vi "machine control.vi"() -> ()   [LabVIEW 2018]
uses:
  ctl/state machine.ctl
  ctl/state machine_read waveform.ctl
  <vilib>/Utility/file.llb/Write To Spreadsheet File (string).vi
panel:
  out "error out":errorcluster
  out "Channel detail information":string[](array[string])
  in  "Convert Y unit to voltage":bool=TRUE
  out "Log":string
  in  "Stop LabVIEW":bool
  out "Last read waveform time(ms)":u32
  in  "Interval(ms)":u32=2000 min=2000 step=100
  in  "Read waveform(continuous)":bool
  in  "CH2":T1
  in  "CH1":T2
  in  "Syntax Testing":cluster{"Syntax":string, "Send":bool}={"Syntax"="*IDN?", "Send"=FALSE}
  in  "Save XY graph":bool
  out "XY Graph":cluster{dbl[], dbl[]}[](graph)
  out "Read buffer":string
  in  "Get instrument information":bool
  in  "Read waveform(single)":bool
  in  "Horizontal scale(TIME/DIV)":T3(ring)
  in  "Autoset":bool
  in  "Device":refnum<visa-resource-name>
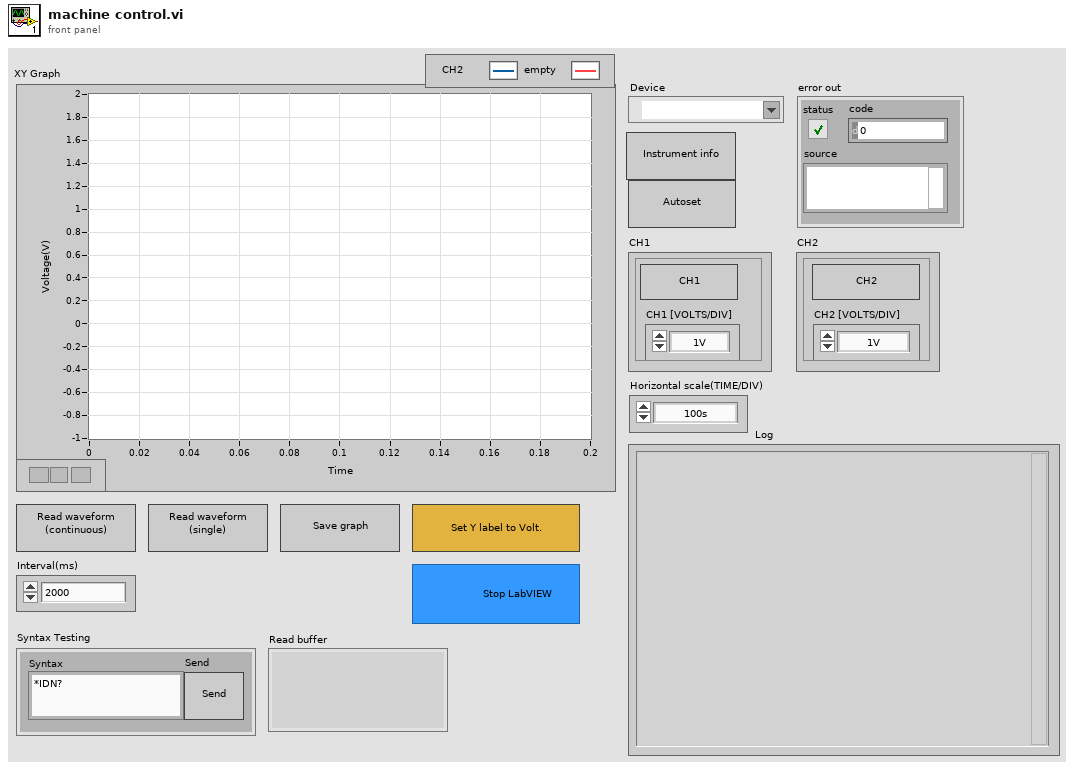
[diagram p1: front panel]
types:
  T1 = cluster{"Enable CH2":bool, "CH2 [VOLTS/DIV]":enum16{"1V", "500mV", "200mV", "100mV", "50mV", "20mV", "10mV", "5mV", "2mV"}}
  T2 = cluster{"Enable CH1":bool, "CH1 [VOLTS/DIV]":enum16{"1V", "500mV", "200mV", "100mV", "50mV", "20mV", "10mV", "5mV", "2mV"}}
  T3 = enum16{"100s", "50s", "20s", "10s", "5s", "2s", "1s", "500ms", "200ms", "100ms", "50ms", "20ms", "10ms", "5ms", "2ms", "1ms", "500£gs", "200£gs ", "100£gs ", "50£gs ", "20£gs ", "10£gs ", "5£gs ", "2£gs", "1£gs", "500ns", "200ns", "100ns", "50ns", "20ns", "10ns", "5ns", "2ns", "1ns"}
  T4 = typedef "state machine.ctl" = enum16{"Initialize", "Open VISA", "Run", "Close VISA"}
  T5 = typedef "state machine_read waveform.ctl" = enum16{"Read waveform", "Data parsing", "Plot graph"}
  T6 = enum16{"1V", "500mV", "200mV", "100mV", "50mV", "20mV", "10mV", "5mV", "2mV"}
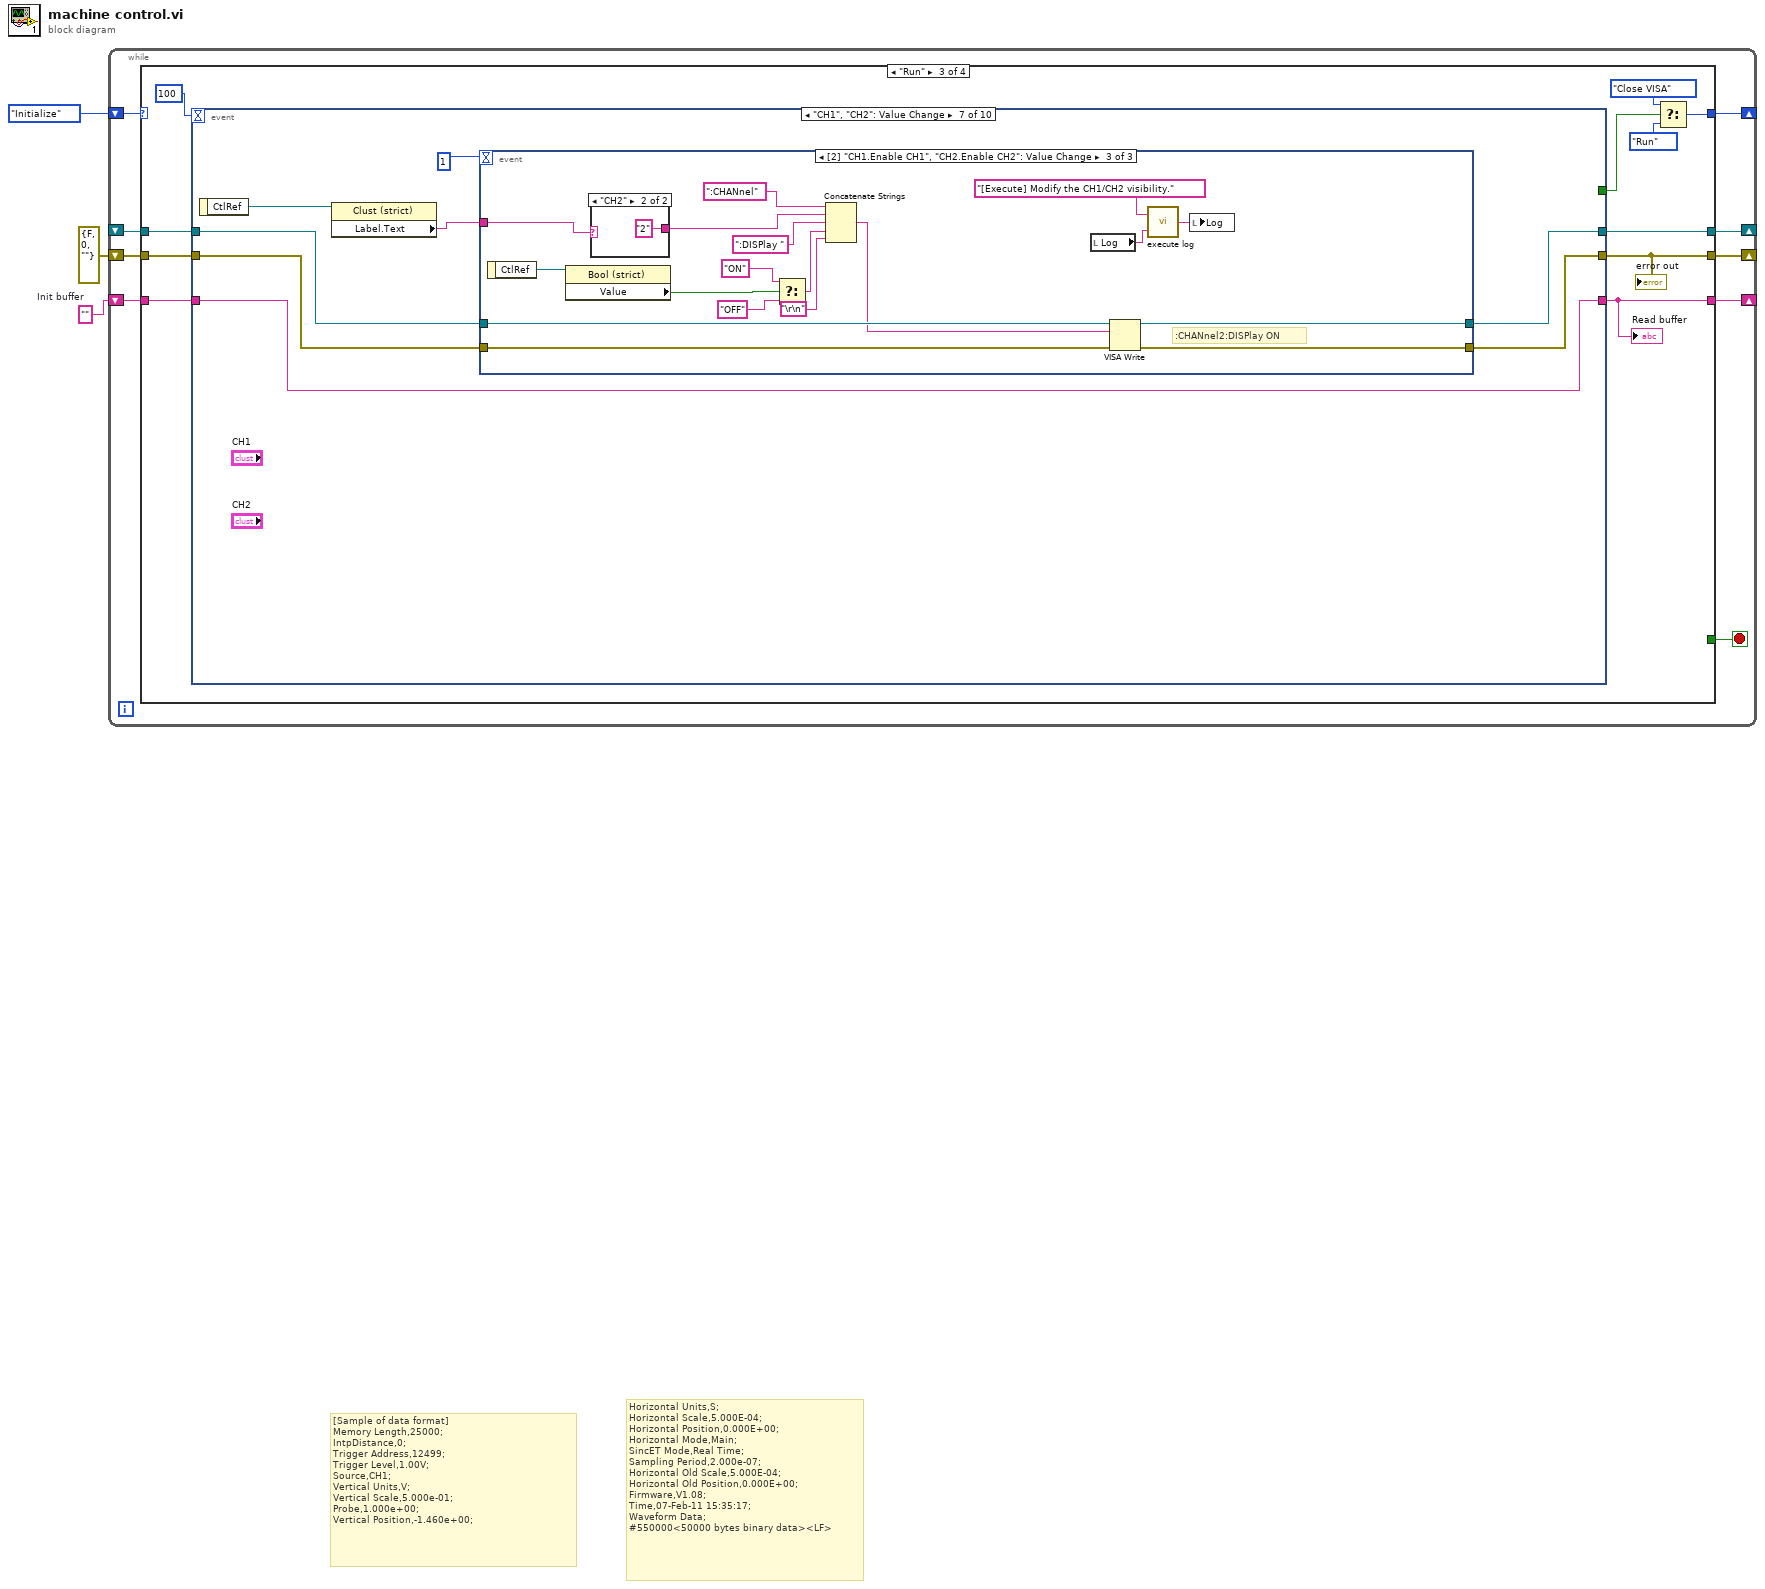
[diagram p0: block diagram]
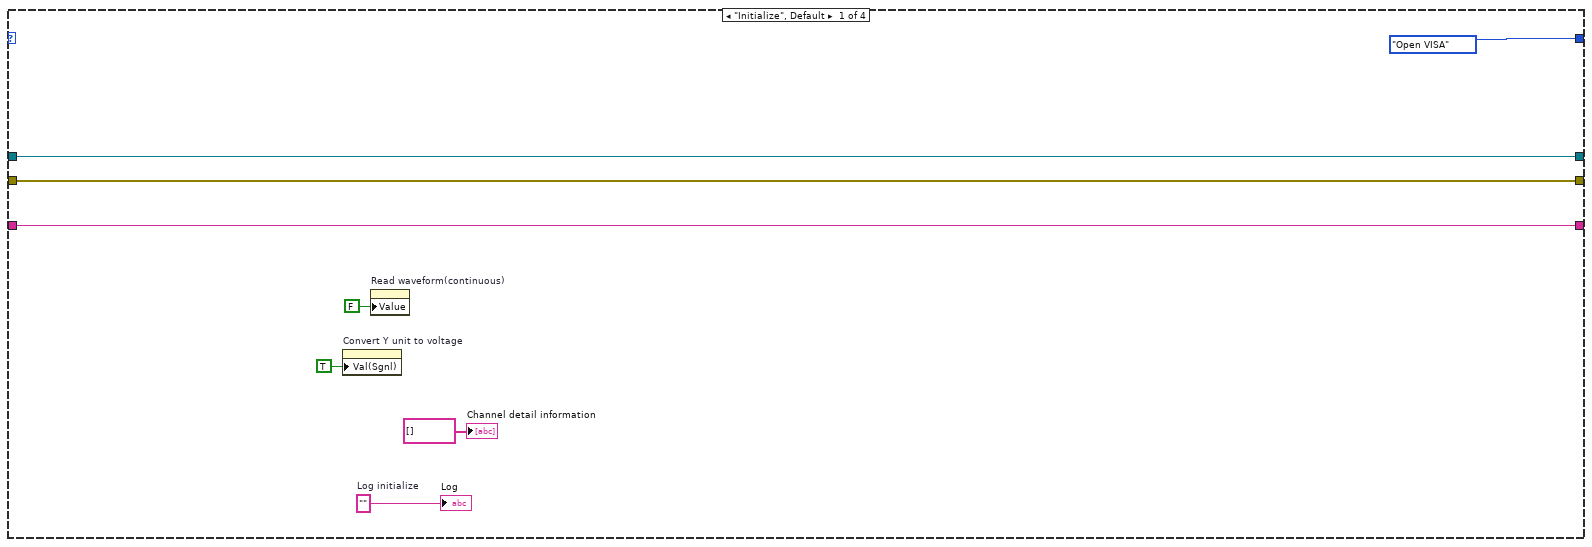
[diagram p2: hidden frame]
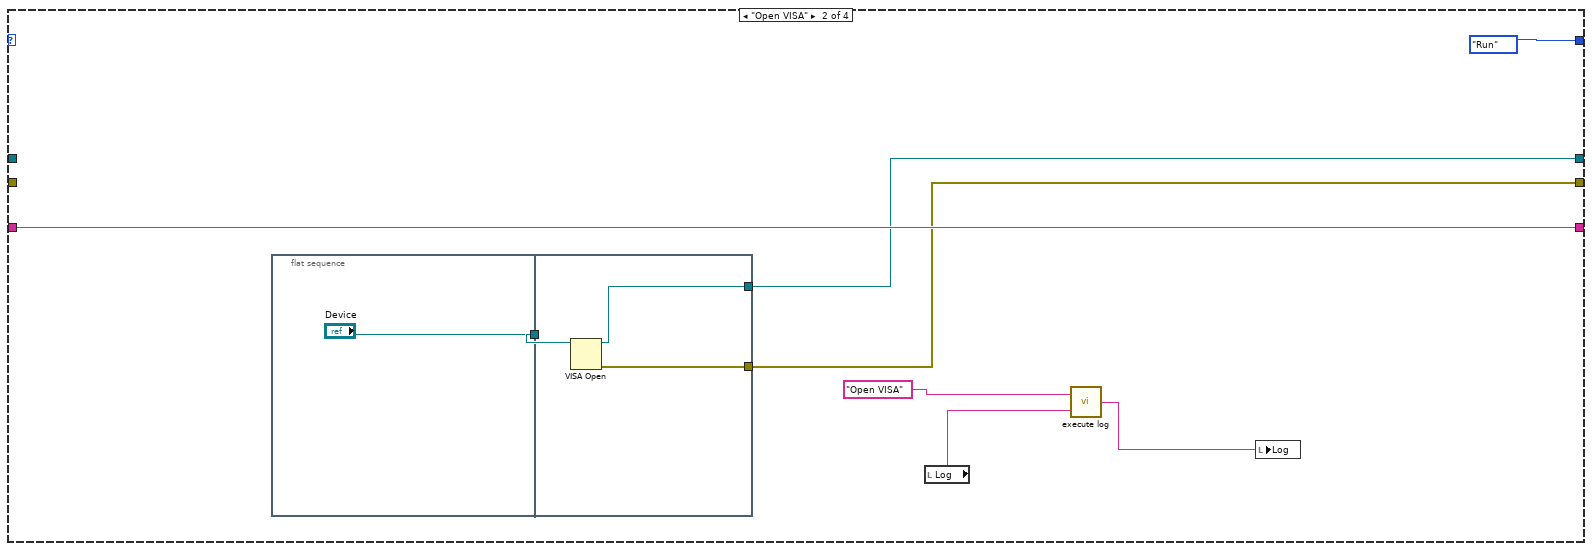
[diagram p3: hidden frame]
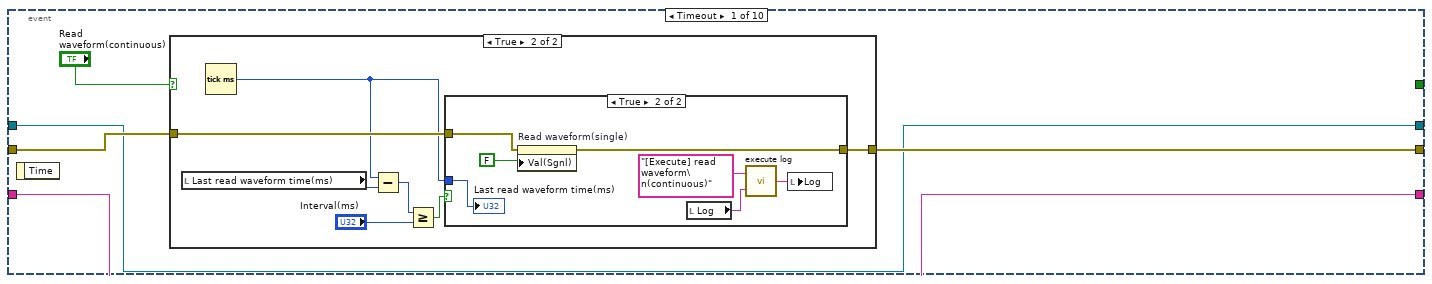
[diagram p4: hidden frame]
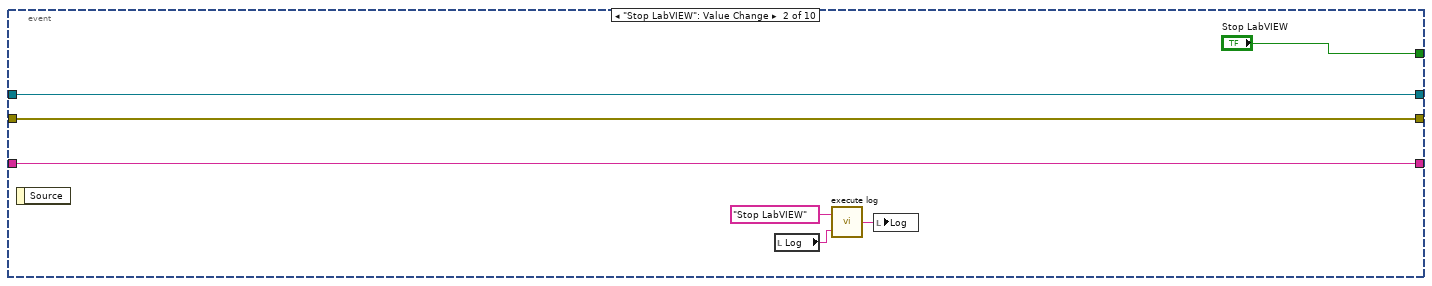
[diagram p7: hidden frame]
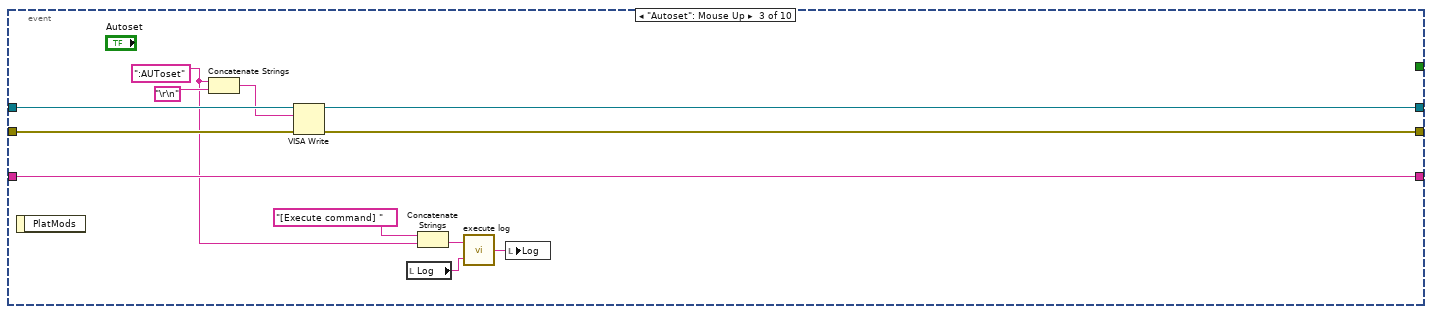
[diagram p8: hidden frame]
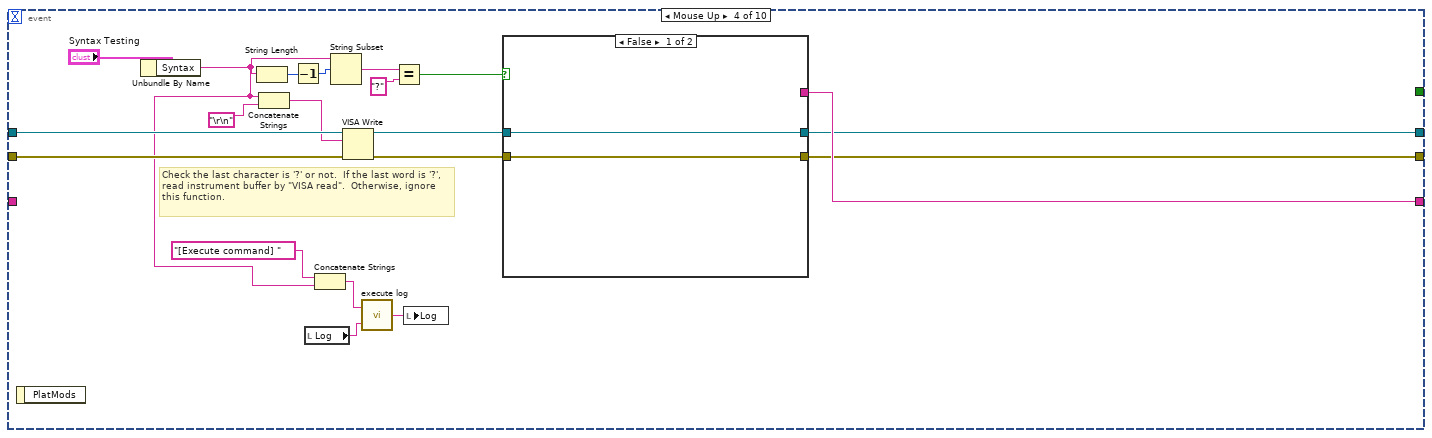
[diagram p9: hidden frame]
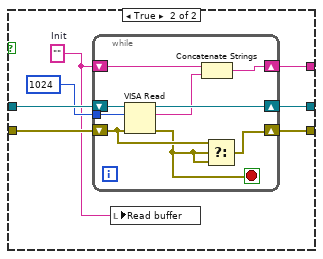
[diagram p10: hidden frame]
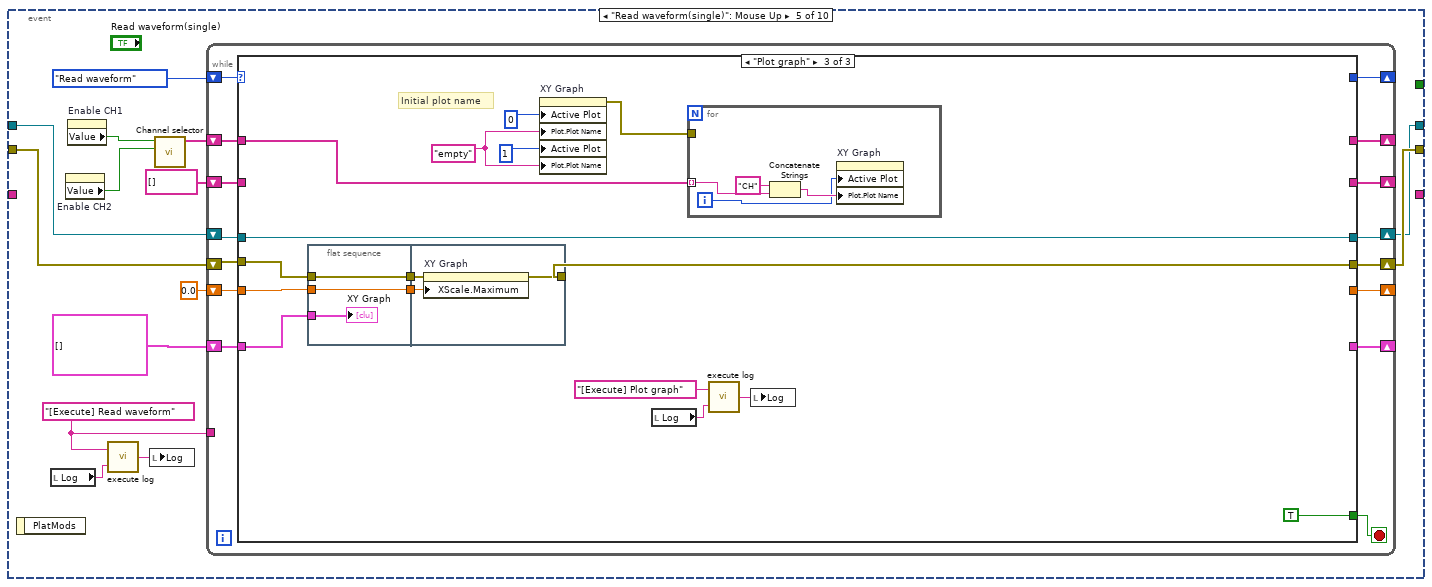
[diagram p11: hidden frame]
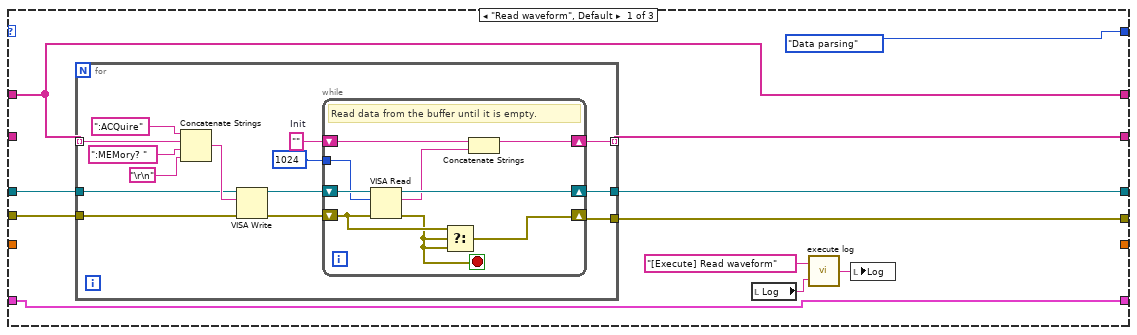
[diagram p12: hidden frame]
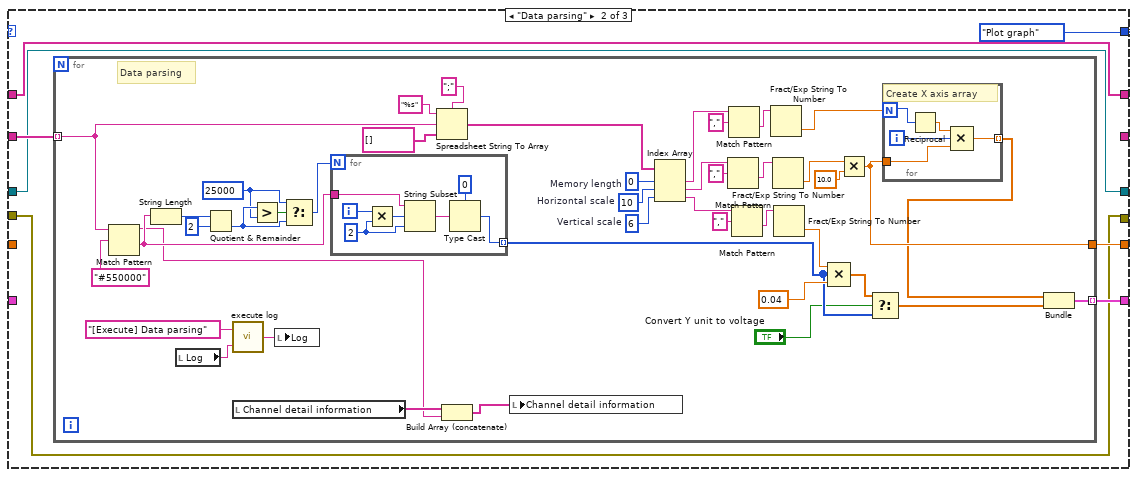
[diagram p13: hidden frame]
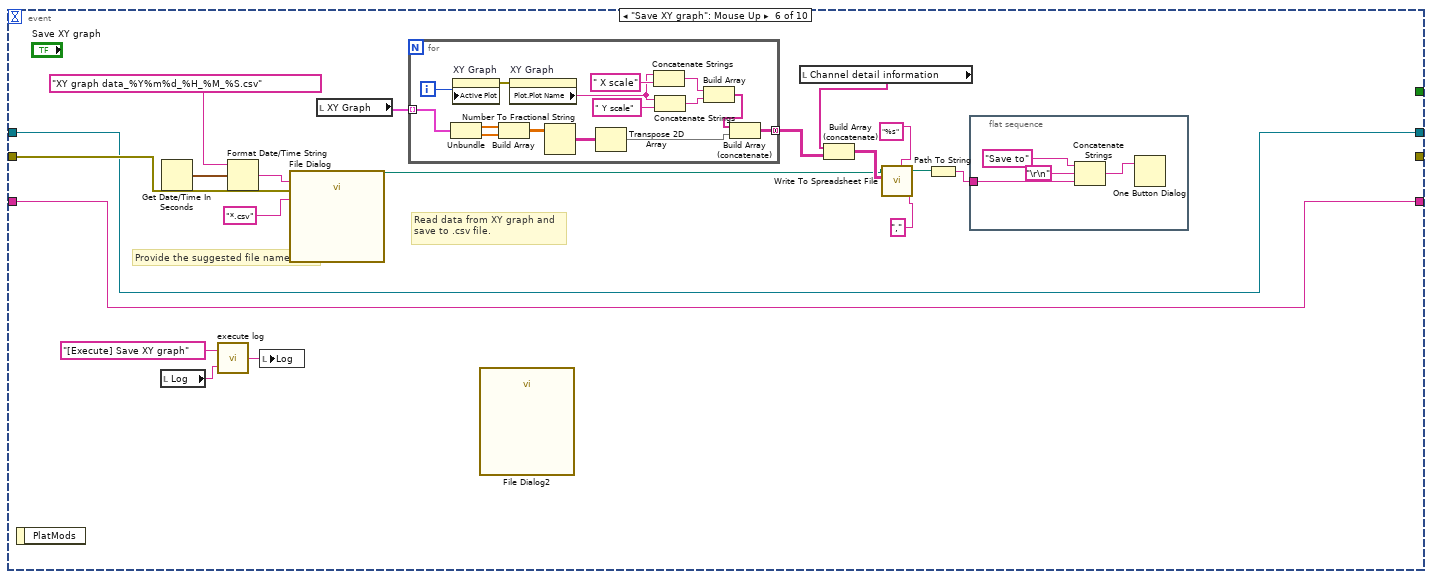
[diagram p14: hidden frame]
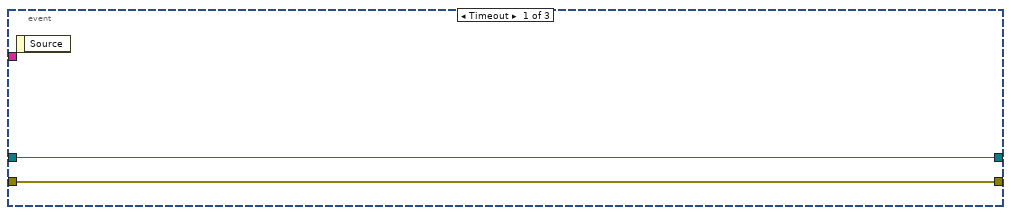
[diagram p15: hidden frame]
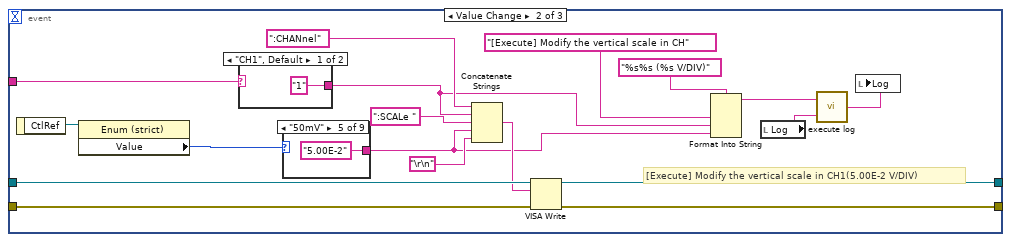
[diagram p16: hidden frame]
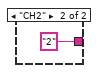
[diagram p17: hidden frame]
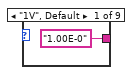
[diagram p18: hidden frame]
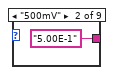
[diagram p19: hidden frame]
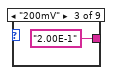
[diagram p20: hidden frame]
diagram:
  w2 = ""  # Init buffer
  # "Horizontal Units,S;\nHorizontal Scale,5.000E-04;\nHorizontal Position,0.000E+00;\nHorizontal Mode,Main;\nSincET Mode,Real Time;\nSampling Period,2.000e-07;\nHorizontal Old Scale,5.000E-04;\nHorizontal Old Position,0.000E+00;\nFirmware,V1.08;\nTime,07-Feb-11 15:35:17;\nWaveform Data;\n#550000<50000 bytes binary data><LF>"
  # "[Sample of data format]\nMemory Length,25000;\nIntpDistance,0;\nTrigger Address,12499;\nTrigger Level,1.00V;\nSource,CH1;\nVertical Units,V;\nVertical Scale,5.000e-01;\nProbe,1.000e+00;\nVertical Position,-1.460e+00;"
  n1 = while {
    shift-right: [w11] -> _
    shift-left: state_machine."Initialize" -> [w12]
    shift-right: [w8] -> _
    shift-left: w2 -> [w5]
    shift-right: [w9] -> _
    shift-left: _ -> [w6]
    shift-right: [w10] -> _
    shift-left: errorcluster {"status"=FALSE, "code"=0, "source"=""} ("error out") -> [w7]
    stop <- w4 stop-if-true
    n2 = case shown="\"Run\"" w12 {
      tunnel: [state_machine."Open VISA" state_machine."Run" w33 _] -> w11
      tunnel: [w17 w21 w43 w442] -> w10
      tunnel: [w18 w22 w42 _] -> w9
      tunnel: [w19 w27 w41 w443] -> w8
      tunnel: w7 -> [w17 _ w40 w444]
      tunnel: w6 -> [w18 _ w39 w445]
      tunnel: w5 -> [w19 w27 w38 w443]
      tunnel: [_ _ _ TRUE] -> w4
      frame "Initialize", Default {
        w14 = ""  # Log initialize
        n3 = property on="Convert Y unit to voltage" class="Bool (strict)"("Val(Sgnl)"=TRUE ("Read waveform(continuous)")) -> ()  [unwired: 2 in, 2 out]
        n4 = property on="Read waveform(continuous)" class="Bool (strict)"("Value"=FALSE ("Read waveform(continuous)")) -> ()  [unwired: 2 in, 2 out]
        "Log" <- w14
        "Channel detail information" <- string[] [] ("Channel detail information")
      }
      frame "Open VISA" {
        n5 = flat-sequence {
          tunnel: ["Device"] -> w23
          tunnel: w23 -> [w32]
          tunnel: [w31] -> w22
          tunnel: [w30] -> w21
          frame #0 {
          }
          frame #1 {
            n6 = VISA Open(VISA resource name=w32) -> (VISA resource name=w31:refnum<visa-resource-name>, error out=w30:errorcluster)  [unwired: 4 in]
          }
        }
        n7 = local read "Log"() -> (w24:string)
        n8 = call "execute log.vi"("log window"=w24, "input string"="Open VISA") -> ("output string"=w25:string)
        n9 = local write "Log"(w25) -> ()
      }
      frame "Run" {
        n10 = event shown="[6] \"CH1\", \"CH2\": Value Change" {
          selector: _ -> [_ _ _ _ _ _ _ _ _ _]
          dyn-events: _ -> [_ _ _ _ _ _ _ _ _ _]
          timeout: 100 -> [_ _ _ _ _ _ _ _ _ _]
          tunnel: w39 -> [w45 w70 w83 w95 w130 w288 w315 w383 w386 w400]
          tunnel: w40 -> [w47 w71 w82 w92 w129 w289 w316 w382 w385 w399]
          tunnel: [w44 w69 w77 w96 _ w290 w311 w377 w384 w394] -> w41
          tunnel: [w45 w70 w81 w94 w124 w288 w318 w379 w386 w398] -> w42
          tunnel: [w46 w71 w80 w93 w125 _ w317 w378 w385 w397] -> w43
          tunnel: [_ "Stop LabVIEW" _ _ _ _ _ _ _ _] -> w36
          tunnel: w38 -> [w44 w69 w77 _ _ w290 w311 _ w384 w394]
          event Timeout {
            n11 = event-data() -> ()  [unwired: 1 in, 1 out]
            n12 = case shown="True" "Read waveform(continuous)" {
              tunnel: w47 -> [w49 w52]
              tunnel: [w49 w51] -> w46
              frame False {
              }
              frame True {
                n13 = local read "Last read waveform time(ms)"() -> (w56:u32)
                n14 = Tick Count (ms)() -> (millisecond timer value=w50:u32)
                n15 = Subtract(x=w50, y=w56) -> (x-y=w53:u32)
                n16 = Greater Or Equal?(x=w53, y="Interval(ms)") -> (x >= y?=w54:bool)
                n17 = case shown="True" w54 {
                  tunnel: w52 -> [w57 w59]
                  tunnel: [w57 w64] -> w51
                  tunnel: w50 -> [_ w60]
                  frame False {
                    # "Nothing"
                  }
                  frame True {
                    n18 = property on="Read waveform(single)" class="Bool (strict)"(error in=w59, "Val(Sgnl)"=FALSE) -> (error out=w64:errorcluster)  [unwired: 1 in, 1 out]
                    n19 = local read "Log"() -> (w61:string)
                    n20 = call "execute log.vi"("log window"=w61, "input string"="[Execute] read waveform\n(continuous)") -> ("output string"=w62:string)
                    n21 = local write "Log"(w62) -> ()
                    "Last read waveform time(ms)" <- w60
                  }
                }
              }
            }
          }
          event "Stop LabVIEW": Value Change {
            n22 = event-data() -> ()  [unwired: 1 in, 1 out]
            n23 = local read "Log"() -> (w65:string)
            n24 = call "execute log.vi"("log window"=w65, "input string"="Stop LabVIEW") -> ("output string"=w66:string)
            n25 = local write "Log"(w66) -> ()
          }
          event "Autoset": Mouse Up {
            w74 = ":AUToset"
            n26 = event-data() -> ()  [unwired: 1 in, 1 out]
            n27 = Concatenate Strings(w74, "\r\n") -> (w79:string)
            n28 = VISA Write(VISA resource name=w83, write buffer=w79, error in (no error)=w82) -> (VISA resource name out=w81:refnum<visa-resource-name>, error out=w80:errorcluster)  [unwired: 1 out]
            n29 = local read "Log"() -> (w75:string)
            n30 = Concatenate Strings("[Execute command] " ("input string"), w74) -> (w72:string)
            n31 = call "execute log.vi"("log window"=w75, "input string"=w72) -> ("output string"=w76:string)
            n32 = local write "Log"(w76) -> ()
          }
          event "Syntax Testing.Send": Mouse Up {
            # "Check the last character is '?' or not.  If the last word is '?', read instrument buffer by \"VISA read\".  Otherwise, ignore this function."
            n33 = event-data() -> ()  [unwired: 1 in, 1 out]
            n34 = Unbundle By Name("Syntax Testing") -> ("Syntax"=w85:string)
            n35 = String Length(string=w85) -> (length=w98:i32)
            n36 = Concatenate Strings(w85, "\r\n") -> (w90:string)
            n37 = Decrement(x=w98) -> (x-1=w99:i32)
            n38 = local read "Log"() -> (w87:string)
            n39 = Concatenate Strings("[Execute command] " ("input string"), w85) -> (w86:string)
            n40 = String Subset(string=w85, offset (0)=w99) -> (substring=w100:string)  [unwired: 1 in]
            n41 = VISA Write(VISA resource name=w95, write buffer=w90, error in (no error)=w92) -> (VISA resource name out=w103:refnum<visa-resource-name>, error out=w102:errorcluster)  [unwired: 1 out]
            n42 = call "execute log.vi"("log window"=w87, "input string"=w86) -> ("output string"=w88:string)
            n43 = Equal?(x=w100, y="?") -> (x = y?=w97:bool)
            n44 = local write "Log"(w88) -> ()
            n45 = case shown="False" w97 {
              tunnel: w103 -> [w105 w112]
              tunnel: [w105 w111] -> w94
              tunnel: w102 -> [w104 w110]
              tunnel: [w104 w109] -> w93
              tunnel: [_ w107] -> w96
              frame False {
              }
              frame True {
                w106 = ""  # Init
                n46 = while {
                  tunnel: u32 1024 ("byte count") -> [w119]
                  shift-right: [w120] -> w111
                  shift-left: w112 -> [w121]
                  shift-right: [w116] -> w109
                  shift-left: w110 -> [w115]
                  shift-right: [w117] -> w107
                  shift-left: w106 -> [w114]
                  stop <- w113 stop-if-true
                  n47 = VISA Read(VISA resource name=w121, byte count=w119, error in (no error)=w115) -> (VISA resource name out=w120:refnum<visa-resource-name>, read buffer=w118:string, error out=w113:errorcluster)  [unwired: 1 out]
                  n48 = Concatenate Strings(w114, w118) -> (w117:string)
                  n49 = Select(t=w115, s=w113, f=w113) -> (s? t:f=w116:errorcluster)
                }
                n50 = local write "Read buffer"(w106) -> ()
              }
            }
          }
          event "Read waveform(single)": Mouse Up {
            w126 = "[Execute] Read waveform" ("input string")
            n51 = event-data() -> ()  [unwired: 1 in, 1 out]
            n52 = local read "Log"() -> (w127:string)
            n53 = property on="Enable CH2" class="Bool (strict)"() -> ("Value"=w131:bool)  [unwired: 2 in, 2 out]
            n54 = property on="Enable CH1" class="Bool (strict)"() -> ("Value"=w132:bool)  [unwired: 2 in, 2 out]
            n55 = call "execute log.vi"("log window"=w127, "input string"=w126) -> ("output string"=w128:string)
            n56 = local write "Log"(w128) -> ()
            n57 = call "Channel selector.vi"("CH2"=w131, "CH1"=w132) -> ("Array"=w123:string[])  [unwired: 9 in]
            n58 = while {
              shift-right: [w141] -> _
              shift-left: state_machine_read_waveform."Read waveform" -> [w150]
              shift-right: [w147] -> w124
              shift-left: w130 -> [w148]
              shift-right: [w146] -> w125
              shift-left: w129 -> [w149]
              shift-right: [w145] -> _
              shift-left: string[] [] -> [w144]
              shift-right: [w143] -> _
              shift-left: cluster{dbl[], dbl[]}[] [] -> [w140]
              shift-right: [w142] -> _
              shift-left: 0.0 -> [w139]
              tunnel: w126 -> [_]
              shift-right: [w136] -> _
              shift-left: w123 -> [w137]
              stop <- w138 stop-if-true
              n59 = case shown="\"Plot graph\"" w150 {
                tunnel: w149 -> [w161 w186 w259]
                tunnel: w148 -> [w160 w187 w255]
                tunnel: [w159 w187 w255] -> w147
                tunnel: [w158 w186 w257] -> w146
                tunnel: [w157 _ _] -> w145
                tunnel: w144 -> [_ w191 _]
                tunnel: [w152 w190 _] -> w143
                tunnel: [_ w189 _] -> w142
                tunnel: [state_machine_read_waveform."Data parsing" state_machine_read_waveform."Plot graph" _] -> w141
                tunnel: w140 -> [w152 _ w262]
                tunnel: w139 -> [_ _ w261]
                tunnel: [_ _ TRUE] -> w138
                tunnel: w137 -> [w151 w185 w247]
                tunnel: [w151 w185 _] -> w136
                frame "Read waveform", Default {
                  n60 = for {
                    tunnel: w161 -> [w167]
                    tunnel: w160 -> [w166]
                    tunnel: [w165] -> w159
                    tunnel: [w164] -> w158
                    tunnel: [w163] -> w157 mode=indexing
                    tunnel: w151 -> [w162] mode=indexing
                    w170 = ""  # Init
                    n61 = Concatenate Strings(":ACQuire", w162, ":MEMory? ", "\r\n") -> (w169:string)
                    n62 = VISA Write(VISA resource name=w166, write buffer=w169, error in (no error)=w167) -> (VISA resource name out=w173:refnum<visa-resource-name>, error out=w172:errorcluster)  [unwired: 1 out]
                    n63 = while {
                      tunnel: u32 1024 ("byte count") -> [w182]
                      shift-right: [w183] -> w165
                      shift-left: w173 -> [w184]
                      shift-right: [w179] -> w164
                      shift-left: w172 -> [w178]
                      shift-right: [w180] -> w163
                      shift-left: w170 -> [w176]
                      stop <- w177 stop-if-true
                      # "Read data from the buffer until it is empty."
                      n64 = VISA Read(VISA resource name=w184, byte count=w182, error in (no error)=w178) -> (VISA resource name out=w183:refnum<visa-resource-name>, read buffer=w181:string, error out=w177:errorcluster)  [unwired: 1 out]
                      n65 = Select(t=w178, s=w177, f=w177) -> (s? t:f=w179:errorcluster)
                      n66 = Concatenate Strings(w176, w181) -> (w180:string)
                    }
                  }
                  n67 = local read "Log"() -> (w154:string)
                  n68 = call "execute log.vi"("log window"=w154, "input string"="[Execute] Read waveform") -> ("output string"=w155:string)
                  n69 = local write "Log"(w155) -> ()
                }
                frame "Data parsing" {
                  n70 = for {
                    tunnel: w191 -> [w211] mode=indexing
                    tunnel: [w210] -> w190 mode=indexing
                    tunnel: [w209] -> w189
                    w207 = 10  # Horizontal scale
                    w208 = 6  # Vertical scale
                    w218 = 0  # Memory length
                    w214 = 25000 ("y")
                    # "Data parsing"
                    n71 = Match Pattern(string=w211, regular expression="#550000") -> (before substring=w192:string, after substring=w224:string)  [unwired: 1 in, 2 out]
                    n72 = String Length(string=w224) -> (length=w223:i32)
                    n73 = local read "Log"() -> (w197:string)
                    n74 = Quotient & Remainder(x=w223, y=2) -> (floor(x/y)=w226:i32)  [unwired: 1 out]
                    n75 = call "execute log.vi"("log window"=w197, "input string"="[Execute] Data parsing") -> ("output string"=w198:string)
                    n76 = local read "Channel detail information"() -> (w194:string[])
                    n77 = Greater?(x=w226, y=w214) -> (0:w225:bool)
                    n78 = local write "Log"(w198) -> ()
                    n79 = Select(t=w214, s=w225, f=w226) -> (s? t:f=w227:i32)
                    n80 = for {
                      N: w227 -> [_]
                      tunnel: w224 -> [w246]
                      tunnel: [w240] -> w200 mode=indexing
                      i -> [w245]
                      w243 = 2 ("length (rest)")
                      n81 = Multiply(x=w245, y=w243) -> (x*y=w244:i32)
                      n82 = String Subset(string=w246, offset (0)=w244, length (rest)=w243) -> (substring=w241:string)
                      n83 = Type Cast(type=i16 0, x=w241) -> (*(type *) &x=w240:i16)
                    }
                    n84 = Spreadsheet String To Array ("Split by ';'")(delimiter (Tab)=";", format string="%s", spreadsheet string=w211, array type (2D Dbl)=string[] [] ("Array")) -> (array=w232:string[])
                    n85 = Build Array (concatenate)(w194, w192) -> (w193:string[])
                    n86 = local write "Channel detail information"(w193) -> ()
                    n87 = Index Array(array=w232, index #1=w218, index #2=w207, index #3=w208) -> (element #1=w233:string, element #2=w206:string, element #3=w205:string)
                    n88 = Match Pattern(string=w206, regular expression=",") -> (after substring=w230:string)  [unwired: 1 in, 3 out]
                    n89 = Match Pattern(string=w233, regular expression=",") -> (after substring=w229:string)  [unwired: 1 in, 3 out]
                    n90 = Match Pattern(string=w205, regular expression=",") -> (after substring=w231:string)  [unwired: 1 in, 3 out]
                    n91 = Fract/Exp String To Number(string=w229) -> (number=w228:dbl)  [unwired: 3 in, 1 out]
                    n92 = Fract/Exp String To Number(string=w230) -> (number=w234:dbl)  [unwired: 3 in, 1 out]
                    n93 = Fract/Exp String To Number(string=w231) -> (number=w204:dbl)  [unwired: 3 in, 1 out]
                    n94 = Compound Arithmetic op=MULTIPLY(w204, w200, 0.04 ("y")) -> (w201:dbl[])
                    n95 = Multiply(x=w234, y=10.0) -> (x*y=w209:dbl)
                    n96 = Select(t=w201, s="Convert Y unit to voltage", f=w200) -> (s? t:f=w202:dbl[])
                    n97 = for {
                      N: w228 -> [w237]
                      tunnel: w209 -> [w238]
                      tunnel: [w239] -> w199 mode=indexing
                      i -> [w235]
                      # "Create X axis array"
                      n98 = Reciprocal(x=w237) -> (1/x=w236:dbl)
                      n99 = Compound Arithmetic op=MULTIPLY(w236, w235, w238) -> (w239:dbl)
                    }
                    n100 = Bundle(w199, w202) -> (w210:cluster{dbl[], dbl[]})  [unwired: 1 in]
                  }
                }
                frame "Plot graph" {
                  w248 = "empty" ("Plot.Plot Name")
                  # "Initial plot name"
                  n101 = flat-sequence {
                    tunnel: w262 -> [w269]
                    tunnel: w261 -> [w268]
                    tunnel: [w268] -> w260
                    tunnel: w259 -> [w267]
                    tunnel: [w267] -> w258
                    tunnel: w260 -> [w272]
                    tunnel: w258 -> [w271]
                    tunnel: [w270] -> w257
                    frame #0 {
                      "XY Graph" <- w269
                    }
                    frame #1 {
                      n102 = property on="XY Graph" class="XYGraph (strict)"(error in=w271, "XScale.Maximum"=w272) -> (error out=w270:errorcluster)  [unwired: 1 in, 1 out]
                    }
                  }
                  n103 = property on="XY Graph" class="XYGraph (strict)"("Active Plot"=u32 0, "Plot.Plot Name"=w248, "Active Plot"=u32 1, "Plot.Plot Name"=w248) -> (error out=w251:errorcluster)  [unwired: 2 in, 1 out]
                  n104 = local read "Log"() -> (w253:string)
                  n105 = for {
                    tunnel: w247 -> [w266] mode=indexing
                    tunnel: w251 -> [_]
                    i -> [w263]
                    n106 = Concatenate Strings("CH" ("string"), w266) -> (w264:string)
                    n107 = property on="XY Graph" class="XYGraph (strict)"("Active Plot"=w263, "Plot.Plot Name"=w264) -> ()  [unwired: 2 in, 2 out]
                  }
                  n108 = call "execute log.vi"("log window"=w253, "input string"="[Execute] Plot graph") -> ("output string"=w254:string)
                  n109 = local write "Log"(w254) -> ()
                }
              }
            }
          }
          event "Save XY graph": Mouse Up {
            # "Read data from XY graph and save to .csv file."
            # "Provide the suggested file name."
            n110 = event-data() -> ()  [unwired: 1 in, 1 out]
            n111 = local read "Log"() -> (w286:string)
            n112 = Get Date/Time In Seconds() -> (seconds since 1Jan1904=w284:timestamp)
            n113 = call "execute log.vi"("log window"=w286, "input string"="[Execute] Save XY graph") -> ("output string"=w287:string)
            n114 = Format Date/Time String(time format string (%c)="XY graph data_%Y%m%d_%H_%M_%S.csv", seconds (now)=w284) -> (date/time string=w282:string)  [unwired: 1 in]
            n115 = local write "Log"(w287) -> ()
            n116 = call "File Dialog"("default name"=w282, "error in"=w289, "pattern (all files)"="*.csv") -> ("selected path"=w276:path)  [unwired: 9 in, 3 out]
            n117 = local read "XY Graph"() -> (w291:cluster{dbl[], dbl[]}[])
            n118 = for {
              tunnel: [w292] -> w273 mode=concatenating
              tunnel: w291 -> [w304] mode=indexing
              i -> [w301]
              n119 = Unbundle(w304) -> (w305:dbl[], w306:dbl[])
              n120 = property on="XY Graph" class="XYGraph (strict)"("Active Plot"=w301) -> (error out=w302:errorcluster)  [unwired: 2 in, 1 out]
              n121 = Build Array(w305, w306) -> (w303:dbl[][])
              n122 = property on="XY Graph" class="XYGraph (strict)"(error in=w302) -> ("Plot.Plot Name"=w298:string)  [unwired: 1 in, 2 out]
              n123 = Number To Fractional String(number=w303) -> (F-format string=w294:string[][])  [unwired: 3 in]
              n124 = Transpose 2D Array(2D array=w294) -> (transposed array=w293:string[][])
              n125 = Concatenate Strings(w298, " X scale" ("string")) -> (w296:string)
              n126 = Concatenate Strings(w298, " Y scale" ("string")) -> (w297:string)
              n127 = Build Array(w296, w297) -> (w295:string[])
              n128 = Build Array (concatenate)(w295, w293) -> (w292:string[][])
            }
            n129 = call "File Dialog2"() -> ()  [unwired: 12 in, 4 out]
            n130 = local read "Channel detail information"() -> (w274:string[])
            n131 = Build Array (concatenate)(w274, w273) -> (w279:string[][])
            n132 = call-poly <vilib>:"Write To Spreadsheet File.vi"("delimiter (\\t)"="," ("delimiter (\\t)"), "format (%s)"="%s" ("string"), "2D data"=w279, "file path (dialog if empty)"=w276) -> ("new file path (Not A Path if cancelled)"=w275:path)  [unwired: 4 in]
            n133 = Path To String(path=w275) -> (string=w280:string)
            n134 = flat-sequence {
              tunnel: w280 -> [w310]
              frame #0 {
                n135 = Concatenate Strings("Save to" ("message"), "\r\n", w310) -> (w307:string)
                n136 = One Button Dialog(message=w307) -> ()  [unwired: 1 in, 1 out]
              }
            }
          }
          event "CH1", "CH2": Value Change {
            n137 = event-data() -> ("CtlRef"=w314:refnum<vi>)  [unwired: 1 in]
            n138 = property class="Clust (strict)"(reference=w314) -> ("Label.Text"=w313:string)  [unwired: 1 in, 2 out]
            n139 = event shown="[2] \"CH1.Enable CH1\", \"CH2.Enable CH2\": Value Change" {
              selector: _ -> [_ _ _]
              dyn-events: _ -> [_ _ _]
              timeout: 1 -> [_ _ _]
              tunnel: [w320 w336 w363] -> w318
              tunnel: [w319 w335 w364] -> w317
              tunnel: w316 -> [w319 w334 w365]
              tunnel: w315 -> [w320 w333 w366]
              tunnel: w313 -> [_ w330 w359]
              event Timeout {
                n140 = event-data() -> ()  [unwired: 1 in, 1 out]
              }
              event "CH1.CH1 [VOLTS/DIV]", "CH2.CH2 [VOLTS/DIV]": Value Change {
                # "[Execute] Modify the vertical scale in CH1(5.00E-2 V/DIV)"
                n141 = event-data() -> ("CtlRef"=w329:refnum<vi>)  [unwired: 1 in]
                n142 = property class="Enum (strict)"(reference=w329) -> ("Value"=w328:T6)  [unwired: 1 in, 2 out]
                n143 = case shown="\"CH1\", Default" w330 {
                  tunnel: ["1" "2"] -> w321
                  frame "CH1", Default {
                  }
                  frame "CH2" {
                  }
                }
                n144 = case shown="\"50mV\"" w328 {
                  tunnel: ["1.00E-0" "5.00E-1" "2.00E-1" "1.00E-1" "5.00E-2" "2.00E-2" "1.00E-2" "5.00E-3" "2.00E-3"] -> w323
                  frame "1V", Default {
                  }
                  frame "500mV" {
                  }
                  frame "200mV" {
                  }
                  frame "100mV" {
                  }
                  frame "50mV" {
                  }
                  frame "20mV" {
                  }
                  frame "10mV" {
                  }
                  frame "5mV" {
                  }
                  frame "2mV" {
                  }
                }
                n145 = Concatenate Strings(":CHANnel", w321, ":SCALe ", w323, "\r\n") -> (w331:string)
                n146 = VISA Write(VISA resource name=w333, write buffer=w331, error in (no error)=w334) -> (VISA resource name out=w336:refnum<visa-resource-name>, error out=w335:errorcluster)  [unwired: 1 out]
                n147 = Format Into String "Format Into String"(format string="%s%s (%s V/DIV)", "[Execute] Modify the vertical scale in CH" ("input string"), w321, w323) -> (resulting string=w324:string)  [unwired: 2 in, 1 out]
                n148 = local read "Log"() -> (w326:string)
                n149 = call "execute log.vi"("log window"=w326, "input string"=w324) -> ("output string"=w327:string)
                n150 = local write "Log"(w327) -> ()
              }
              event "CH1.Enable CH1", "CH2.Enable CH2": Value Change {
                # ":CHANnel2:DISPlay ON"
                n151 = event-data() -> ("CtlRef"=w367:refnum<vi>)  [unwired: 1 in]
                n152 = property class="Bool (strict)"(reference=w367) -> ("Value"=w350:bool)  [unwired: 1 in, 2 out]
                n153 = case shown="\"CH2\"" w359 {
                  tunnel: ["1" ("string") "2" ("string")] -> w357
                  frame "CH1", Default {
                  }
                  frame "CH2" {
                  }
                }
                n154 = Select(t="ON" ("string"), s=w350, f="OFF" ("string")) -> (s? t:f=w358:string)
                n155 = Concatenate Strings(":CHANnel" ("string"), w357, ":DISPlay " ("string"), w358, "\r\n") -> (w355:string)
                n156 = local read "Log"() -> (w353:string)
                n157 = VISA Write(VISA resource name=w366, write buffer=w355, error in (no error)=w365) -> (VISA resource name out=w363:refnum<visa-resource-name>, error out=w364:errorcluster)  [unwired: 1 out]
                n158 = call "execute log.vi"("log window"=w353, "input string"="[Execute] Modify the CH1/CH2 visibility.") -> ("output string"=w354:string)
                n159 = local write "Log"(w354) -> ()
              }
            }
          }
          event "Get instrument information": Mouse Up {
            n160 = event-data() -> ()  [unwired: 1 in, 1 out]
            n161 = Concatenate Strings("*IDN?" ("input string"), "\r\n") -> (w373:string)
            n162 = VISA Write(VISA resource name=w383, write buffer=w373, error in (no error)=w382) -> (VISA resource name out=w380:refnum<visa-resource-name>, error out=w381:errorcluster)  [unwired: 1 out]
            n163 = VISA Read(VISA resource name=w380, byte count=u32 1024, error in (no error)=w381) -> (VISA resource name out=w379:refnum<visa-resource-name>, read buffer=w377:string, error out=w378:errorcluster)  [unwired: 1 out]
            n164 = local read "Log"() -> (w371:string)
            n165 = call "execute log.vi"("log window"=w371, "input string"="[Execute] Get instrument information.") -> ("output string"=w372:string)
            n166 = local write "Log"(w372) -> ()
          }
          event "Convert Y unit to voltage": Value Change {
            n167 = event-data() -> ()  [unwired: 1 in, 1 out]
            n168 = local read "Convert Y unit to voltage"() -> (w389:bool)
            n169 = Select(t="Voltage(V)" ("regular expression"), s=w389, f="Count" ("regular expression")) -> (s? t:f=w390:string)
            n170 = property on="XY Graph" class="XYGraph (strict)"("YScale.NameLbl.Text"=w390) -> ()  [unwired: 2 in, 2 out]
          }
          event "Horizontal scale(TIME/DIV)": Value Change {
            n171 = event-data() -> ()  [unwired: 1 in, 1 out]
            n172 = case shown="\"5ns\"" "Horizontal scale(TIME/DIV)" {
              tunnel: ["10" "5" "2e-6" "1" "500e-3" "200e-3" "100e-3" "50e-3" "20e-3" "1e-6 " "500e-9" "200e-9" "100e-9" "50e-9" "20e-9" "10e-9" "5e-9" "2e-9" "1e-9" "2" "10e-3" "5e-3" "2e-3" "1e-3" "500e-6" "200e-6" "100e-6" "50e-6" "20e-6" "10e-6" "5e-6" "20" "50" "100"] -> w401
              frame "10s", Default {
              }
              frame "5s" {
              }
              frame "2£gs" {
              }
              frame "1s" {
              }
              frame "500ms" {
              }
              frame "200ms" {
              }
              frame "100ms" {
              }
              frame "50ms" {
              }
              frame "20ms" {
              }
              frame "1£gs" {
              }
              frame "500ns" {
              }
              frame "200ns" {
              }
              frame "100ns" {
              }
              frame "50ns" {
              }
              frame "20ns" {
              }
              frame "10ns" {
              }
              frame "5ns" {
              }
              frame "2ns" {
              }
              frame "1ns" {
              }
              frame "2s" {
              }
              frame "10ms" {
              }
              frame "5ms" {
              }
              frame "2ms" {
              }
              frame "1ms" {
              }
              frame "500£gs" {
              }
              frame "200£gs " {
              }
              frame "100£gs " {
              }
              frame "50£gs " {
              }
              frame "20£gs " {
              }
              frame "10£gs " {
              }
              frame "5£gs " {
              }
              frame "20s" {
              }
              frame "50s" {
              }
              frame "100s" {
              }
            }
            n173 = Concatenate Strings(":TIMebase:SCALe ", w401, "\r\n") -> (w396:string)
            n174 = VISA Write(VISA resource name=w400, write buffer=w396, error in (no error)=w399) -> (VISA resource name out=w398:refnum<visa-resource-name>, error out=w397:errorcluster)  [unwired: 1 out]
            n175 = local read "Log"() -> (w392:string)
            n176 = call "execute log.vi"("log window"=w392, "input string"="[Execute]Modify horizontal scale.") -> ("output string"=w393:string)
            n177 = local write "Log"(w393) -> ()
          }
        }
        "Read buffer" <- w41
        "error out" <- w43
        n178 = Select(t=state_machine."Close VISA", s=w36, f=state_machine."Run") -> (s? t:f=w33:T4)
      }
      frame "Close VISA" {
        n179 = local read "Log"() -> (w439:string)
        n180 = call "execute log.vi"("log window"=w439, "input string"="[Execute] Close VISA") -> ("output string"=w440:string)
        n181 = local write "Log"(w440) -> ()
        n182 = VISA Close(VISA resource name=w445, error in (no error)=w444) -> (error out=w442:errorcluster)
      }
    }
  }
